vi "Proportional Stabilization 2.0.vi"() -> ()   [LabVIEW 2013]
uses:
  Global Variables/Global Stop.vi
panel:
  out "Thin Etalon Pos Setp on Activation":i32
  in  "Thin Etalon Position Setpoint":i32
  in  "Etalon Selection":enum16{"Thick Etalon", "Thin Etalon"}(ring)
  in  "Activate Output":bool
  out "Thick Etalon Pos Setp on Activation":i32
  out "Wavenumber on Activation":dbl format="%.4f"
  in  "Correction Output":bool
  out "correction steps":dbl
  in  "Difference Threshold":dbl=0.019999999999999997
  in  "Proportional Correction Factor":dbl=300.0
  out "New Wavemeter Value":bool
  out "Out of Range":bool
  in  "Stop":bool
  out "Loop Counter":i32
  in  "Thick Etalon Position Setpoint":i32
  in  "Invert Output":bool
  in  "Wavenumber Setpoint":dbl format="%.4f"
  out "Wavenumber Acquisition":dbl format="%.4f"
  # "Invert Output\nif moving beyond\nFlash Position"
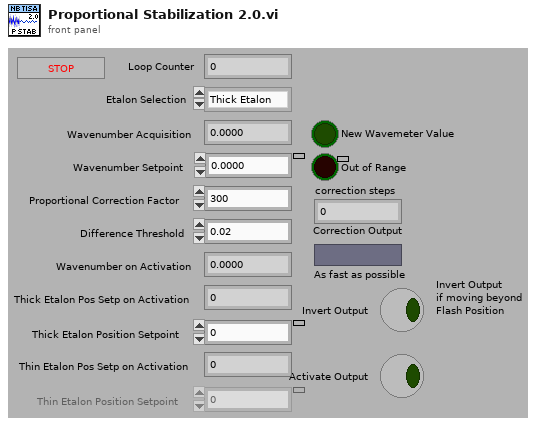
[diagram p1: front panel]
types:
  T1 = enum8{"Enabled", "Disabled", "Disabled and Grayed Out"}
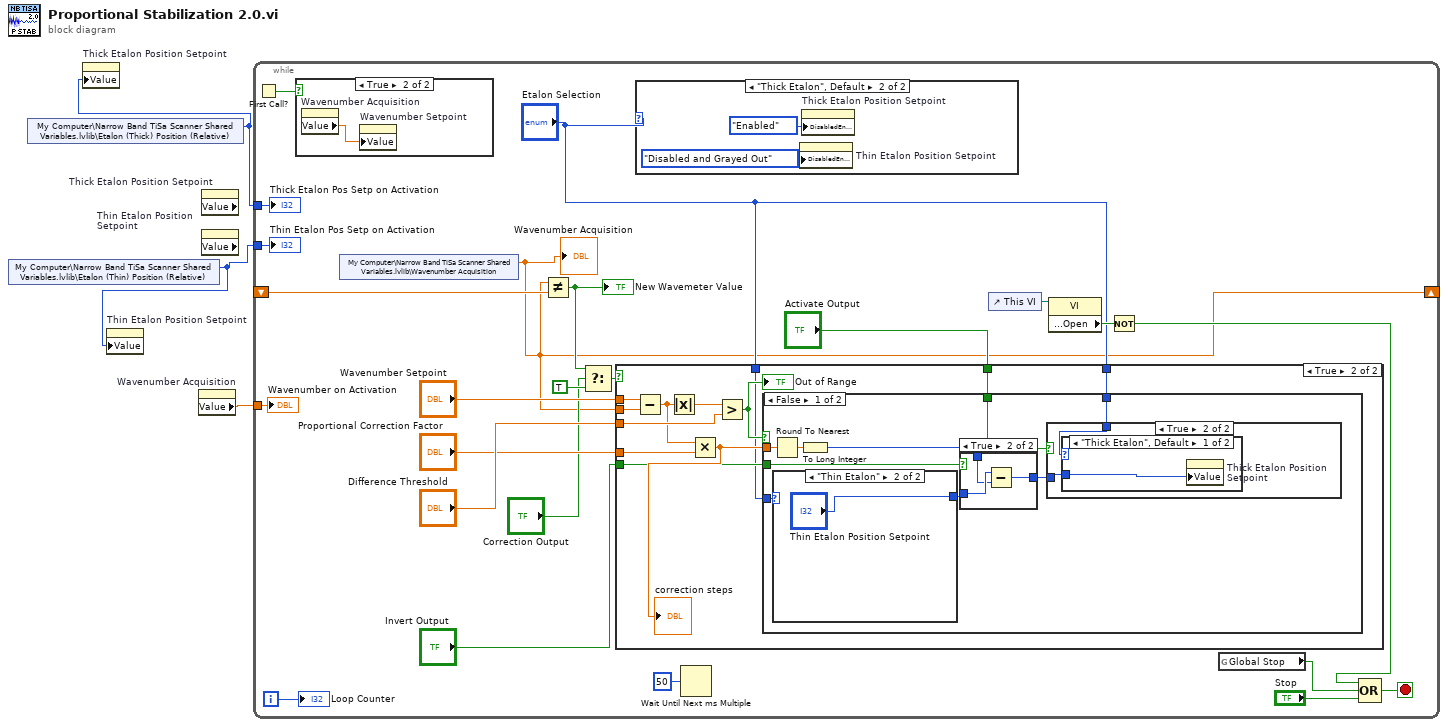
[diagram p0: block diagram]
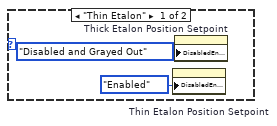
[diagram p2: hidden frame]
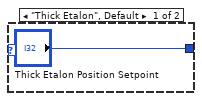
[diagram p4: hidden frame]
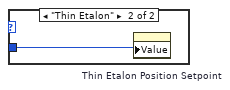
[diagram p6: hidden frame]
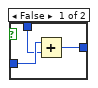
[diagram p7: hidden frame]
diagram:
  n1 = shared-variable "My Computer\\Narrow Band TiSa Scanner Shared Variables.lvlib\\Etalon (Thin) Position (Relative)"() -> (w1:i32)  [unwired: 1 in, 1 out]
  n2 = shared-variable "My Computer\\Narrow Band TiSa Scanner Shared Variables.lvlib\\Etalon (Thick) Position (Relative)"() -> (w2:i32)  [unwired: 1 in, 1 out]
  n3 = property on="Thick Etalon Position Setpoint" class="DigNum (strict)"("Value"=w2) -> ()  [unwired: 2 in, 2 out]
  n4 = property on="Thin Etalon Position Setpoint" class="DigNum (strict)"("Value"=w1) -> ()  [unwired: 2 in, 2 out]
  n5 = property on="Wavenumber Acquisition" class="DigNum (strict)"() -> ("Value"=w3:dbl)  [unwired: 2 in, 2 out]
  n6 = property on="Thick Etalon Position Setpoint" class="DigNum (strict)" props=["Value"]() -> ()  [unwired: 2 in, 3 out]
  n7 = property on="Thin Etalon Position Setpoint" class="DigNum (strict)" props=["Value"]() -> ()  [unwired: 2 in, 3 out]
  n8 = while {
    shift-right: [w4] -> _
    shift-left: _ -> [w26]
    tunnel: w3 -> [w9]
    tunnel: w2 -> [w8]
    tunnel: w1 -> [w6]
    i -> [w23]
    stop <- w13 stop-if-true
    n9 = First Call?() -> (First Call?: T/F=w27:bool)
    n10 = case shown="True" w27 {
      frame False {
      }
      frame True {
        n11 = property on="Wavenumber Acquisition" class="DigNum (strict)"() -> ("Value"=w65:dbl)  [unwired: 2 in, 2 out]
        n12 = property on="Wavenumber Setpoint" class="DigNum (strict)"("Value"=w65) -> ()  [unwired: 2 in, 2 out]
      }
    }
    n13 = shared-variable "My Computer\\Narrow Band TiSa Scanner Shared Variables.lvlib\\Wavenumber Acquisition"() -> (w4:dbl)  [unwired: 1 in, 1 out]
    "Wavenumber Acquisition" <- w4
    n14 = Not Equal?(x=w4, y=w26) -> (x != y?=w18:bool)
    "New Wavemeter Value" <- w18
    n15 = Select(t=w18, s="Correction Output", f=TRUE) -> (s? t:f=w19:bool)
    n16 = case shown="True" w19 {
      tunnel: "Wavenumber Setpoint" -> [_ w43]
      tunnel: w4 -> [_ w42]
      tunnel: "Difference Threshold" -> [_ w39]
      tunnel: "Proportional Correction Factor" -> [_ w37]
      tunnel: "Invert Output" -> [_ w35]
      tunnel: "Activate Output" -> [_ w34]
      tunnel: "Etalon Selection" -> [_ w33]
      tunnel: "Etalon Selection" -> [_ w32]
      frame False {
      }
      frame True {
        n17 = Subtract(x=w43, y=w42) -> (x-y=w38:dbl)
        n18 = Absolute Value(x=w38) -> (abs(x)=w41:dbl)
        n19 = Multiply(x=w38, y=w37) -> (x*y=w36:dbl)
        "correction steps" <- w36
        n20 = Greater?(x=w41, y=w39) -> (0:w40:bool)
        "Out of Range" <- w40
        n21 = case shown="False" w40 {
          tunnel: w36 -> [w51 _]
          tunnel: w35 -> [w49 _]
          tunnel: w34 -> [w46 _]
          tunnel: w33 -> [w45 _]
          tunnel: w32 -> [w44 _]
          frame False {
            n22 = Round To Nearest(number=w51) -> (nearest integer value=w48:dbl)
            n23 = case shown="\"Thin Etalon\"" w44 {
              tunnel: ["Thick Etalon Position Setpoint" "Thin Etalon Position Setpoint"] -> w52
              frame "Thick Etalon", Default {
              }
              frame "Thin Etalon" {
              }
            }
            n24 = To Long Integer(number=w48) -> (32bit integer=w47:i32)
            n25 = case shown="True" w49 {
              tunnel: w52 -> [w61 w64]
              tunnel: w47 -> [w60 w63]
              tunnel: [w59 w62] -> w50
              frame False {
                n26 = Add(x=w61, y=w60) -> (x+y=w59:i32)
              }
              frame True {
                n27 = Subtract(x=w64, y=w63) -> (x-y=w62:i32)
              }
            }
            n28 = case shown="True" w46 {
              tunnel: w50 -> [_ w56]
              tunnel: w45 -> [_ w55]
              frame False {
              }
              frame True {
                n29 = case shown="\"Thick Etalon\", Default" w55 {
                  tunnel: w56 -> [w57 w58]
                  frame "Thick Etalon", Default {
                    n30 = property on="Thick Etalon Position Setpoint" class="DigNum (strict)"("Value"=w57) -> ()  [unwired: 2 in, 2 out]
                  }
                  frame "Thin Etalon" {
                    n31 = property on="Thin Etalon Position Setpoint" class="DigNum (strict)"("Value"=w58) -> ()  [unwired: 2 in, 2 out]
                  }
                }
              }
            }
          }
          frame True {
          }
        }
      }
    }
    n32 = case shown="\"Thick Etalon\", Default" "Etalon Selection" {
      frame "Thin Etalon" {
        n33 = property on="Thin Etalon Position Setpoint" class="DigNum (strict)"("DisabledEnum"=T1."Enabled" ("Disabled")) -> ()  [unwired: 2 in, 2 out]
        n34 = property on="Thick Etalon Position Setpoint" class="DigNum (strict)"("DisabledEnum"=T1."Disabled and Grayed Out" ("Disabled")) -> ()  [unwired: 2 in, 2 out]
      }
      frame "Thick Etalon", Default {
        n35 = property on="Thin Etalon Position Setpoint" class="DigNum (strict)"("DisabledEnum"=T1."Disabled and Grayed Out" ("Disabled")) -> ()  [unwired: 2 in, 2 out]
        n36 = property on="Thick Etalon Position Setpoint" class="DigNum (strict)"("DisabledEnum"=T1."Enabled" ("Disabled")) -> ()  [unwired: 2 in, 2 out]
      }
    }
    n37 = Wait Until Next ms Multiple(millisecond multiple=u32 50) -> ()  [unwired: 1 out]
    n38 = control-ref of="This VI"() -> (w14:refnum<vi>)
    n39 = property class="VI"(reference=w14) -> ("Front Panel.Open"=w15:bool)  [unwired: 1 in, 2 out]
    n40 = Not(x=w15) -> (.not. x?=w12:bool)
    n41 = global read "Global Stop.vi" "Global Stop"() -> (w11:bool)
    n42 = Compound Arithmetic op=OR(w12, w11, "Stop") -> (w13:bool)
    "Loop Counter" <- w23
    "Wavenumber on Activation" <- w9
    "Thick Etalon Pos Setp on Activation" <- w8
    "Thin Etalon Pos Setp on Activation" <- w6
  }
